vi "Set.vi"(6 "abort (F)":bool, 8 "element":bool, 11 "TagData in":refnum<class "TagData.lvclass">) -> (0 "previous element":bool, 1 "sequence":u64, 3 "TagData out":refnum<class "TagData.lvclass">, 4 "aborted?":bool)   [LabVIEW 2020, in "Tag-bool.lvlib" / "TagData.lvclass"]
uses:
  <extravilib>/ChannelInstances/Tag-bool/TagData.lvclass
  <extravilib>/ChannelInstances/Tag-bool/TagData.lvclass/TagData.ctl
  <resource>/ChannelSupport/_ChannelSupport/_ChannelSupport.lvlib
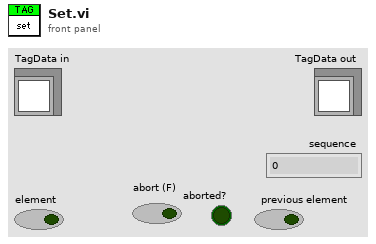
[diagram p1: front panel]
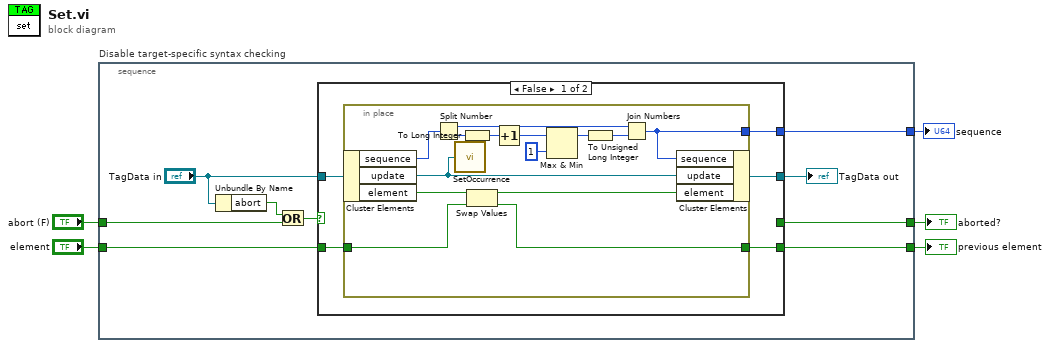
[diagram p0: block diagram]
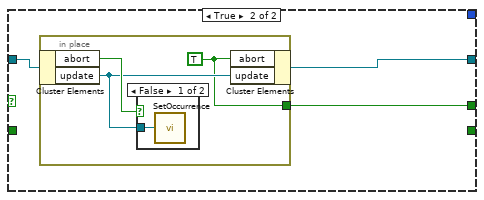
[diagram p2: hidden frame]
diagram:
  n1 = stacked-sequence "Disable target-specific syntax checking" {
    tunnel: "element" -> [w13]
    tunnel: [w12] -> w4
    tunnel: "abort (F)" -> [w9]
    tunnel: [w7] -> w2
    tunnel: [w6] -> w1
    frame #0 {
      n2 = Unbundle By Name("TagData in") -> ("abort"=w10:bool)
      n3 = Or(x=w10, y=w9) -> (x .or. y?=w8:bool)
      n4 = case shown="False" w8 {
        tunnel: [w19 w34] -> w14
        tunnel: w13 -> [w18 _]
        tunnel: [w17 _] -> w12
        tunnel: "TagData in" -> [w16 w36]
        tunnel: [_ w35] -> w7
        tunnel: [w15 _] -> w6
        frame False {
          n5 = in-place {
            in-place-border: w18 -> [w31]
            in-place-border: [w21] -> w17
            in-place-border: [w29] -> w15
            n6 = in-place-cluster #1(w16) -> ("sequence"=w22:u64, "update"=w30:refnum<k4>, "element"=w33:bool)
            n7 = Split Number(x=w22) -> (hi(x)=w23:u32, lo(x)=w27:u32)
            n8 = call <resource>:"SetOccurrence.vi"("occurrence"=w30) -> ()  [unwired: 9 in]
            n9 = To Long Integer(number=w27) -> (32bit integer=w25:i32)
            n10 = Swap Values(12:w33, 14:w31) -> (1:w32:bool, 3:w29:bool)  [unwired: 1 in]
            n11 = Increment(x=w25) -> (x+1=w28:i32)
            n12 = Max & Min(x=w28, y=1) -> (max(x,y)=w26:i32)  [unwired: 1 out]
            n13 = To Unsigned Long Integer(number=w26) -> (unsigned 32bit integer=w24:u32)
            n14 = Join Numbers(hi=w23, lo=w24) -> ((hi.lo)=w21:u64)
            n15 = in-place-cluster #1("sequence"=w21, "update"=w30, "element"=w32) -> (w19:refnum<class "TagData.lvclass">)
          }
        }
        frame True {
          n16 = in-place {
            in-place-border: [w37] -> w35
            w37 = TRUE ("abort")
            n17 = in-place-cluster #2(w36) -> ("abort"=w39:bool, "update"=w38:refnum<k4>)
            n18 = case shown="False" w39 {
              tunnel: w38 -> [w40 _]
              frame False {
                n19 = call <resource>:"SetOccurrence.vi"("occurrence"=w40) -> ()  [unwired: 9 in]
              }
              frame True {
              }
            }
            n20 = in-place-cluster #2("abort"=w37, "update"=w38) -> (w34:refnum<class "TagData.lvclass">)
          }
        }
      }
      "TagData out" <- w14
    }
  }
  "sequence" <- w4
  "aborted?" <- w2
  "previous element" <- w1
